vi "Recurse.vi"(6 "Error":errorcluster, 10 "Message":refnum<class "Message.lvclass">, 11 "Actor":refnum<class "Actor.lvclass">) -> (2 "Message":refnum<class "Message.lvclass">, 3 "Actor":refnum<class "Actor.lvclass">, 4 "Error":errorcluster)   [LabVIEW 2020, in "_Template.lvlib" / "{{Message}}.lvlib"]
uses:
  {{Message}}.lvlib
  Message/Message.lvclass
  jettl/jettl/Actor/Actor.lvclass
panel:
  # "This front panel should not be manipulated."
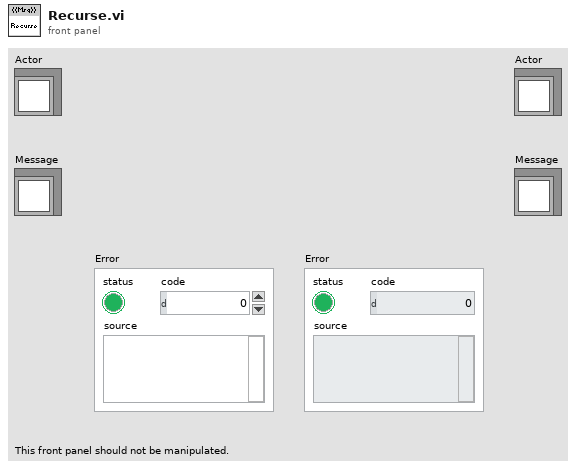
[diagram p1: front panel]
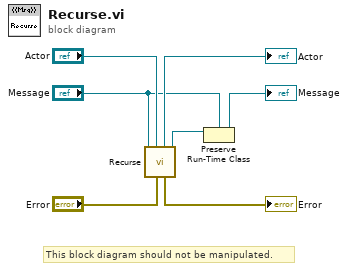
[diagram p0: block diagram]
diagram:
  # "This block diagram should not be manipulated."
  n1 = call-dynamic "Recurse.vi"("Error"="Error", "Actor"="Actor", "Message"="Message") -> ("Message"=w3:refnum<class "Message.lvclass">, "Error"=→"Error":errorcluster, "Actor"=→"Actor":refnum<class "Actor.lvclass">)  [unwired: 6 in]
  n2 = Preserve Run-Time Class(object in=w3, 2:"Message") -> (object out=→"Message":refnum<class "Message.lvclass">)  [unwired: 1 in, 1 out]
